vi "Init User Search.vi"(8 "error in (no error)":errorcluster, 11 "[V] User List in":refnum<class "[V] User List.lvclass">) -> (0 "error out":errorcluster, 3 "[V] User List out":refnum<class "[V] User List.lvclass">)   [LabVIEW 2020, in "[V] User List.lvlib" / "[V] User List.lvclass"]
uses:
  [V] User List.lvclass
  [V] User List.lvclass/[V] User List.ctl
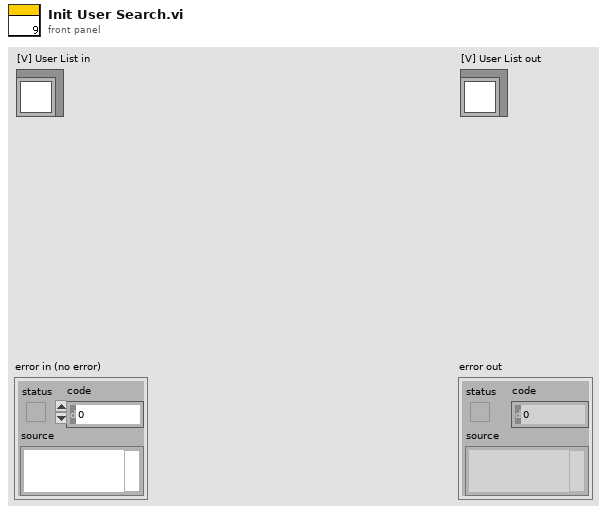
[diagram p1: front panel]
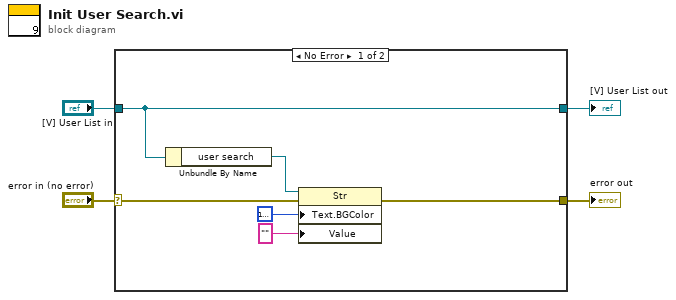
[diagram p0: block diagram]
diagram:
  n1 = case shown="No Error" "error in (no error)" {
    selector: "error in (no error)" -> [w7 w12]
    tunnel: [w5 w12] -> w3
    tunnel: [w10 w11] -> w1
    tunnel: "[V] User List in" -> [w10 w11]
    frame No Error {
      n2 = Unbundle By Name(w10) -> ("user search"=w8:refnum<vi>)
      n3 = property on="Property Node" class="Str"(reference=w8, error in=w7, "Text.BGColor"=u32 16777216, "Value"="") -> (error out=w5:errorcluster)  [unwired: 1 out]
    }
    frame Error {
    }
  }
  "error out" <- w3
  "[V] User List out" <- w1
